vi "Draw Rotated Robot.vi"(8 "offset":cluster{"left":i32, "top":i32}={"left"=100, "top"=100}, 9 "YPR (deg)":cluster{"yaw":dbl, "pitch":dbl, "roll":dbl} {"yaw" format="%.1g"; "pitch" format="%.1g"; "roll" format="%.1g"}, 11 "Picture in":picture) -> (3 "picture out":picture)   [LabVIEW 2025]
uses:
  <vilib>/robotics/Kinematics/RotateX.vi
  <vilib>/robotics/Kinematics/RotateY.vi
  <vilib>/robotics/Kinematics/RotateZ.vi
  <vilib>/Analysis/baseanly.llb/A x B.vi
  <vilib>/Analysis/baseanly.llb/Real A x B.vi
  <vilib>/robotics/Kinematics/NI_Kinematics.lvlib
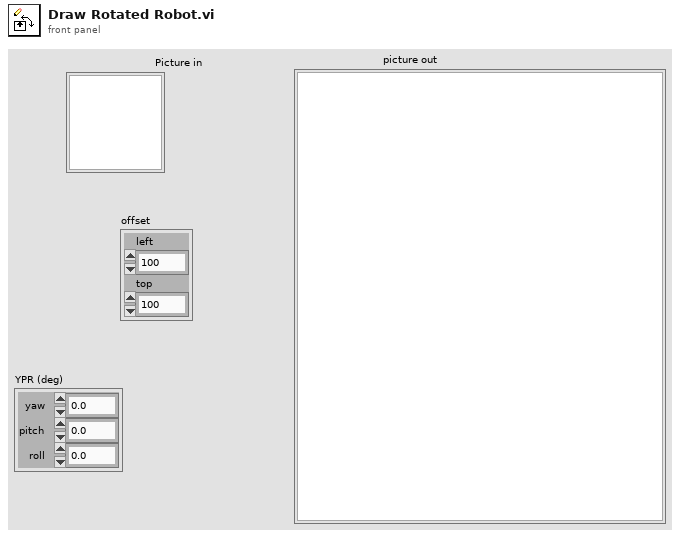
[diagram p1: front panel]
types:
  T1 = cluster{"horizontal":enum16{"left", "center", "right"}, "vertical":enum16{"top", "center", "bottom"}}
  T2 = typedef "NI_Matrix.lvlib/RealMatrix.ctl" = dbl[][]
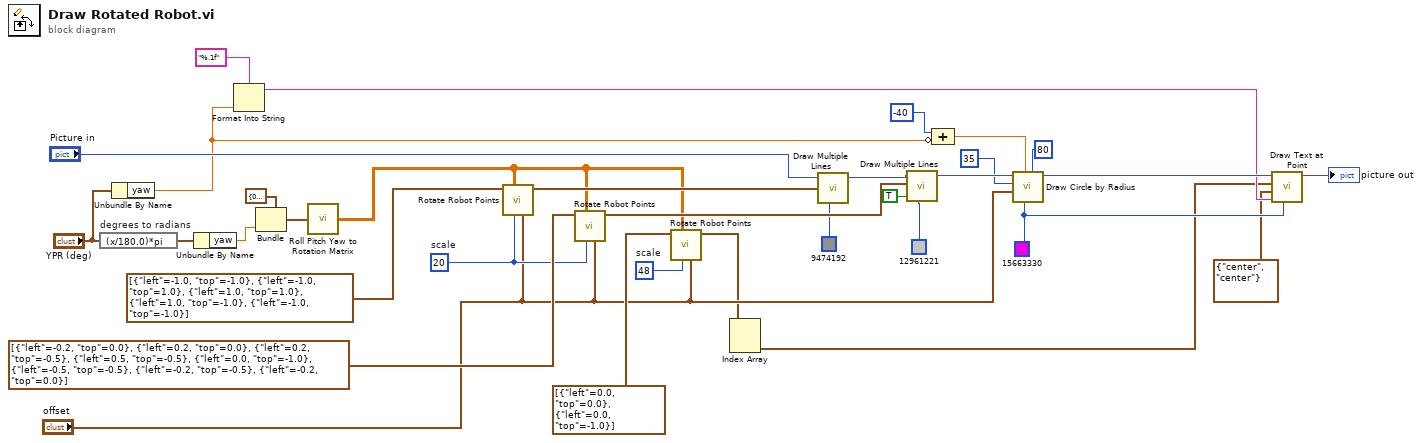
[diagram p0: block diagram]
diagram:
  w4 = 48  # scale
  w9 = u32 15663330 ("color(black)")
  w27 = 20  # scale
  n1 = expression code="(x/180.0)*pi" "degrees to radians"("YPR (deg)") -> (w32:cluster{"yaw":dbl, "pitch":dbl, "roll":dbl})
  n2 = Unbundle By Name("YPR (deg)") -> ("yaw"=w11:dbl)
  n3 = Unbundle By Name(w32) -> ("yaw"=w16:dbl)
  n4 = Format Into String(format string="%.1f", w11) -> (resulting string=w10:string)  [unwired: 2 in, 1 out]
  n5 = Bundle(cluster=cluster{"roll":dbl, "pitch":dbl, "yaw":dbl} {"roll"=0.0, "pitch"=0.0, "yaw"=0.0} ("angles"), "yaw"=w16) -> (w31:cluster{"roll":dbl, "pitch":dbl, "yaw":dbl})  [unwired: 2 in]
  n6 = call <vilib>:"Roll Pitch Yaw to Rotation Matrix.vi"("angles"=w31) -> ("rotation matrix"=w6:T2)
  n7 = call "Rotate Robot Points.vi"("ofst"="offset", "scale"=w27, "rotation matrix"=w6, "Array in"=cluster{"left":dbl, "top":dbl}[] [{"left"=-1.0, "top"=-1.0}, {"left"=-1.0, "top"=1.0}, {"left"=1.0, "top"=1.0}, {"left"=1.0, "top"=-1.0}, {"left"=-1.0, "top"=-1.0}]) -> ("Array out"=w26:cluster{dbl, dbl}[])  [unwired: 7 in]
  n8 = call "Rotate Robot Points.vi"("ofst"="offset", "scale"=w27, "rotation matrix"=w6, "Array in"=cluster{"left":dbl, "top":dbl}[] [{"left"=-0.2, "top"=0.0}, {"left"=0.2, "top"=0.0}, {"left"=0.2, "top"=-0.5}, {"left"=0.5, "top"=-0.5}, {"left"=0.0, "top"=-1.0}, {"left"=-0.5, "top"=-0.5}, {"left"=-0.2, "top"=-0.5}, {"left"=-0.2, "top"=0.0}]) -> ("Array out"=w24:cluster{dbl, dbl}[])  [unwired: 7 in]
  n9 = call "Rotate Robot Points.vi"("ofst"="offset", "scale"=w4, "rotation matrix"=w6, "Array in"=cluster{"left":dbl, "top":dbl}[] [{"left"=0.0, "top"=0.0}, {"left"=0.0, "top"=-1.0}]) -> ("Array out"=w2:cluster{dbl, dbl}[])  [unwired: 7 in]
  n10 = Index Array(array=w2) -> (element #2=w1:cluster{dbl, dbl})  [unwired: 2 in, 1 out]
  n11 = call <vilib>:"Draw Multiple Lines.vi"("picture"="Picture in", "line endpoints"=w26, "color(black)"=u32 9474192) -> ("new picture"=w25:picture)  [unwired: 6 in]
  n12 = call <vilib>:"Draw Multiple Lines.vi"("picture"=w25, "line endpoints"=w24, "fill?(F)"=TRUE, "color(black)"=u32 12961221) -> ("new picture"=w20:picture)  [unwired: 5 in]
  n13 = Compound Arithmetic op=ADD(i16 -40 ("start angle(0)"), invert w11) -> (w15:dbl)
  n14 = call <vilib>:"Draw Circle by Radius.vi"("arc size(360)"=i16 80, "color(black)"=w9, "start angle(0)"=w15, "pixel center"="offset", "radius"=35, "picture"=w20) -> ("new picture"=w13:picture)  [unwired: 5 in]
  n15 = call <vilib>:"Draw Text at Point.vi"("text color(black)"=w9, "text"=w10, "alignment(left, top)"=T1 {"horizontal"=enum."center", "vertical"=enum."center"}, "origin"=w1, "picture"=w13) -> ("new picture"=→"picture out":picture)  [unwired: 5 in, 1 out]
